vi "Save_Data.vi"(8 "error in (no error)":errorcluster, 11 "Message Queues out":T1) -> (0 "error out":errorcluster)   [LabVIEW 2023]
uses:
  Message Queue/All Message Queues.ctl
  Message Queue/Message Cluster.ctl
  controls/UI Data.ctl
  Drivers/Resideo Gas Valve/Type Definitions/Vesta Info.ctl
  Drivers/Resideo Gas Valve/Type Definitions/Temperature Control.ctl
  controls/Timer Application Cluster.ctl
  controls/Burner Duty Cycle.ctl
  Hybrid Water Heater/Type Definitions/HEWH MW100 Data Cluster.ctl
  Hybrid Water Heater/Custom Instrument Control/MW100/Type Definitions/HEWH Module 4 Relay Status.ctl
  Message Queue/Enqueue Message (Single).vi
  Message Queue/Message Queue.lvlib
panel:
  in  "Debug":bool
  out "Debug":string[](array[string])
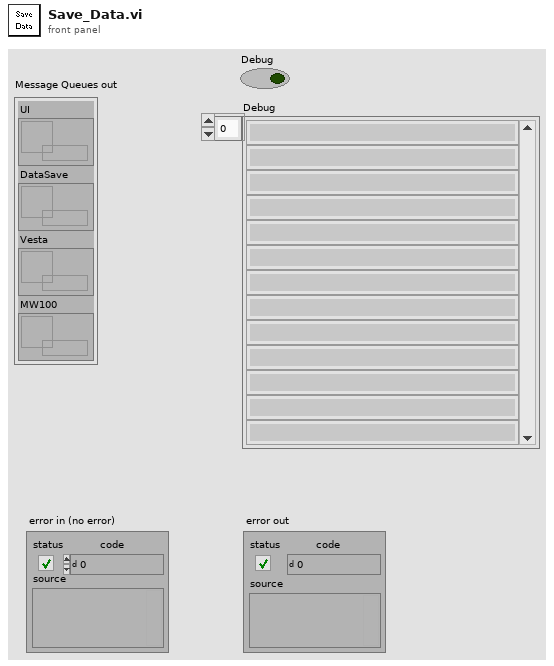
[diagram p1: front panel]
types:
  T1 = typedef "Message Queue.lvlib/All Message Queues.ctl" = cluster{"UI":refnum<queue>, "DataSave":refnum<queue>, "Vesta":refnum<queue>, "MW100":refnum<queue>}
  T2 = typedef "UI Data.ctl" = cluster{"Vesta Data Output":T3, "VestaTemperature":T4, "Timer Application Data":T5, "Data Array":string[][], "MW Output":T7}
  T3 = typedef "Vesta Info.ctl" = cluster{"Temp_W_Raw_U":u16, "Temp_W_Raw_L":u16, "Temperature Water (F)":dbl, "Temperature Water Compensated (F)":dbl, "Temperature Ambient (F)":dbl, "Setpoint Location (F)":dbl, "Heat Request":string, "Fault Ram":string, "PWM DCDC Value":u16, "Pilot Voltage (mV)":dbl, "Setpoint Actual (F)":dbl, "Differential Actual (F)":dbl, "Setpoint User (F)":dbl, "Differential User (F)":dbl, "Termperature FIltered -TCO (F)":dbl, "Temp_C_Raw_1 - Sensor Voltage":string, "Temp_C_Raw_2 - Sensor Voltage":string, "Chamber Sensor Temperature (F)":dbl, "LDO Base Temperature (F)":dbl, "LDO Timer (sec)":i16, "Disabled (0)":bool, "Warming (1)":bool, "Heating (2)":bool, "Cooling Data Write (3)":bool, "Cooling (4)":bool, "Data Read (5)":bool, "N/A":bool, "Temperature Trip (7)":bool, "Burner":bool}
  T4 = typedef "Temperature Control.ctl" = cluster{"Water Heater Temp (°F)":u16, "Differential  (°F)":dbl}
  T5 = typedef "Timer Application Cluster.ctl" = cluster{"Duty Cycle":T6}
  T6 = typedef "Burner Duty Cycle.ctl" = cluster{"Burner ON Time (Seconds)":dbl, "Burner OFF Time (Seconds)":dbl, "Main Burner Flag":bool, "Burner Power Mode":u8}
  T7 = typedef "HEWH MW100 Data Cluster.ctl" = cluster{"TC1-Channel 021":dbl, "TC2-Channel 022":dbl, "TC3-Channel 023":dbl, "TC4-Channel 024":dbl, "TC5-Channel 025":dbl, "TC6-Channel 026":dbl, "TC7-Channel 017":dbl, "TC8-Channel 028":dbl, "TC9-Channel 029":dbl, "TC10-Channel 030":dbl, "TC Tree Average":dbl, "TC DWN- Channel 027":dbl, "RTDin-Channel 031":dbl, "RTDout-Channel 032":dbl, "RTDamb-Channel 033":dbl, "PSI1-Channel 011":dbl, "PSI2-Channel 012":dbl, "PSI3-Channel 013":dbl, "PSI4-Channel 014":dbl, "UE State-Channel 015":dbl, "LE State-Channel 016":dbl, "Module 4 Relay Status Output":T8}
  T8 = typedef "HEWH Module 4 Relay Status.ctl" = cluster{"INTELLIFAUCET TEMP(T)/FLOW(F) (CH 041)":bool, "INTELLIFAUCET READY (CH 042)":bool, "INTELLIFAUCET START (CH 043)":bool, "INTELLIFAUCET STOP (CH 044)":bool, "MAIN POWER RELAY (CH 047)":bool, "NOT USED (CH 045)":bool, "NOT USED (CH 046)":bool, "PURGE VALVE RELAY (CH 048)":bool, "OUTLET VALVE RELAY (CH 049)":bool, "INLET VALVE RELAY (CH 050)":bool, "Intellifaucet (% Open)":dbl, "Proportioning Valve (%Open)":dbl, "Intellifaucet Temp Setpoint (F)":dbl}
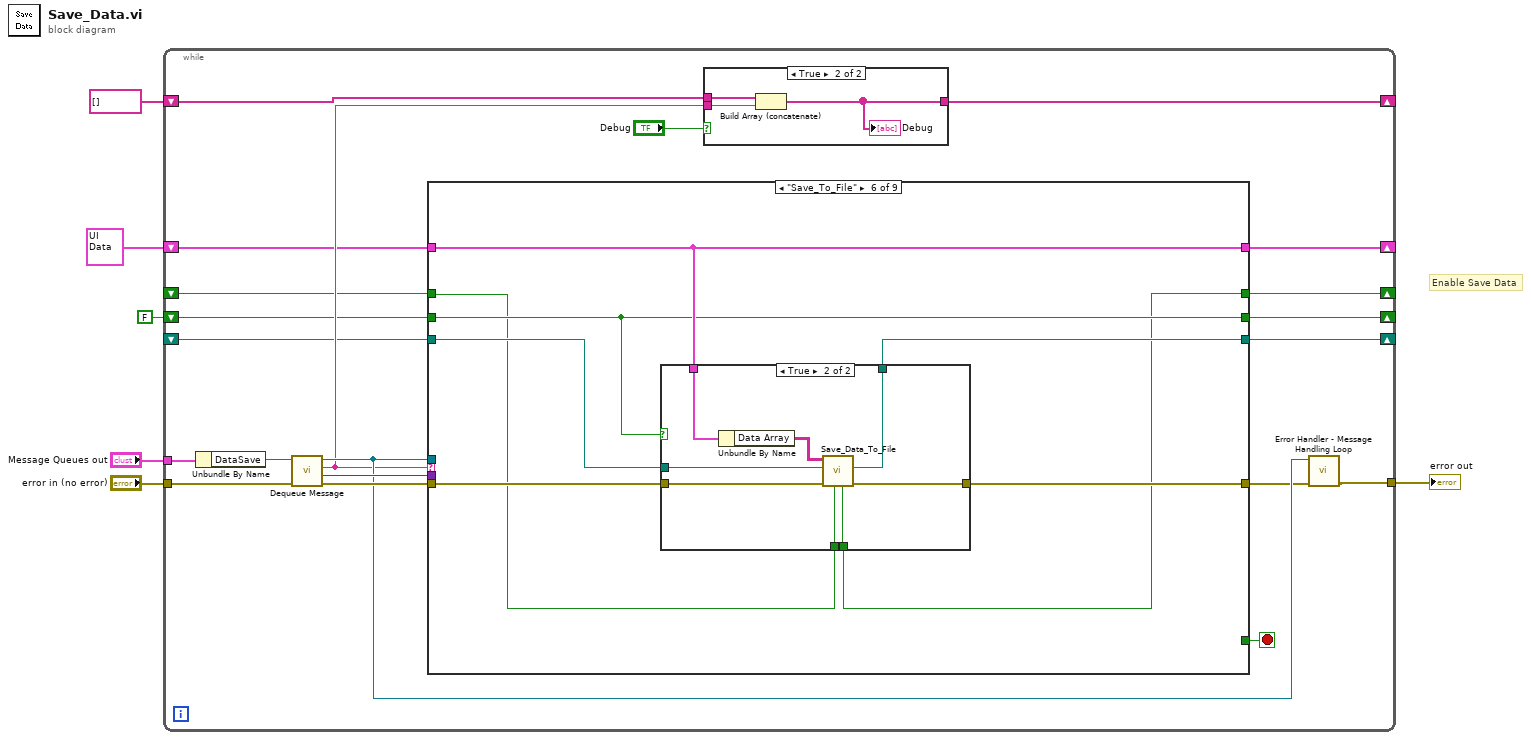
[diagram p0: block diagram]
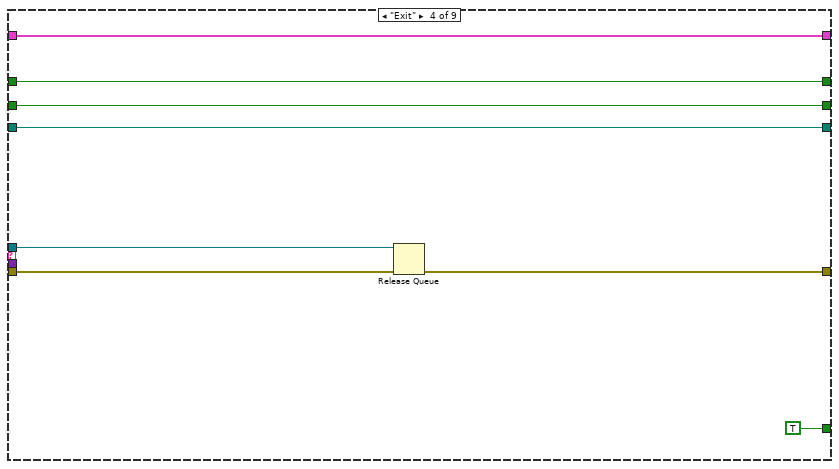
[diagram p6: hidden frame]
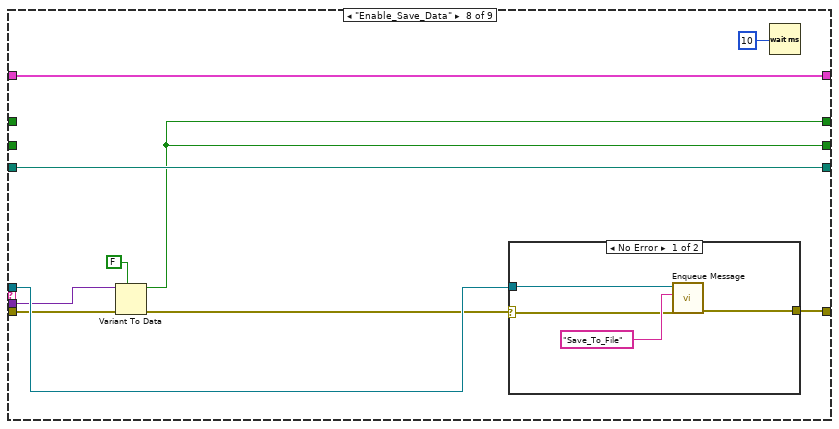
[diagram p10: hidden frame]
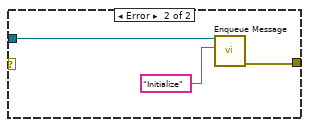
[diagram p11: hidden frame]
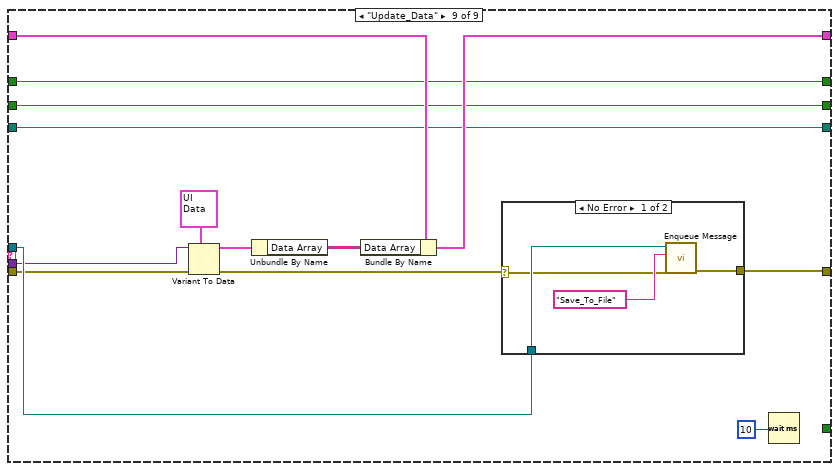
[diagram p12: hidden frame]
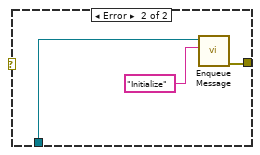
[diagram p13: hidden frame]
diagram:
  # "Enable Save Data"
  n1 = while {
    tunnel: "Message Queues out" -> [w20]
    tunnel: "error in (no error)" -> [w24]
    tunnel: [w17] -> w3
    shift-right: [w21] -> _
    shift-left: string[] [] -> [w22]
    shift-right: [w13] -> _
    shift-left: T2 {"Vesta Data Output"={"Temp_W_Raw_U"=0, "Temp_W_Raw_L"=0, "Temperature Water (F)"=0.0, "Temperature Water Compensated (F)"=0.0, "Temperature Ambient (F)"=0.0, "Setpoint Location (F)"=0.0, "Heat Request"="", "Fault Ram"="", "PWM DCDC Value"=0, "Pilot Voltage (mV)"=0.0, "Setpoint Actual (F)"=0.0, "Differential Actual (F)"=0.0, "Setpoint User (F)"=0.0, "Differential User (F)"=0.0, "Termperature FIltered -TCO (F)"=0.0, "Temp_C_Raw_1 - Sensor Voltage"="", "Temp_C_Raw_2 - Sensor Voltage"="", "Chamber Sensor Temperature (F)"=0.0, "LDO Base Temperature (F)"=0.0, "LDO Timer (sec)"=0, "Disabled (0)"=FALSE, "Warming (1)"=FALSE, "Heating (2)"=FALSE, "Cooling Data Write (3)"=FALSE, "Cooling (4)"=FALSE, "Data Read (5)"=FALSE, "N/A"=FALSE, "Temperature Trip (7)"=FALSE, "Burner"=FALSE}, "VestaTemperature"={"Water Heater Temp (°F)"=135, "Differential  (°F)"=10.0}, "Timer Application Data"={"Duty Cycle"={"Burner ON Time (Seconds)"=60.0, "Burner OFF Time (Seconds)"=60.0, "Main Burner Flag"=FALSE, "Burner Power Mode"=0}}, "Data Array"=[], "MW Output"={"TC1-Channel 021"=0.0, "TC2-Channel 022"=0.0, "TC3-Channel 023"=0.0, "TC4-Channel 024"=0.0, "TC5-Channel 025"=0.0, "TC6-Channel 026"=0.0, "TC7-Channel 017"=0.0, "TC8-Channel 028"=0.0, "TC9-Channel 029"=0.0, "TC10-Channel 030"=0.0, "TC Tree Average"=0.0, "TC DWN- Channel 027"=0.0, "RTDin-Channel 031"=0.0, "RTDout-Channel 032"=0.0, "RTDamb-Channel 033"=0.0, "PSI1-Channel 011"=0.0, "PSI2-Channel 012"=0.0, "PSI3-Channel 013"=0.0, "PSI4-Channel 014"=0.0, "UE State-Channel 015"=0.0, "LE State-Channel 016"=0.0, "Module 4 Relay Status Output"={"INTELLIFAUCET TEMP(T)/FLOW(F) (CH 041)"=FALSE, "INTELLIFAUCET READY (CH 042)"=FALSE, "INTELLIFAUCET START (CH 043)"=FALSE, "INTELLIFAUCET STOP (CH 044)"=FALSE, "MAIN POWER RELAY (CH 047)"=FALSE, "NOT USED (CH 045)"=FALSE, "NOT USED (CH 046)"=FALSE, "PURGE VALVE RELAY (CH 048)"=FALSE, "OUTLET VALVE RELAY (CH 049)"=FALSE, "INLET VALVE RELAY (CH 050)"=FALSE, "Intellifaucet (% Open)"=0.0, "Proportioning Valve (%Open)"=0.0, "Intellifaucet Temp Setpoint (F)"=0.0}}} ("Data Cluster Output") -> [w14]
    shift-right: [w12] -> _
    shift-left: FALSE -> [w11]
    shift-right: [w10] -> _
    shift-left: _ -> [w9]
    shift-right: [w8] -> _
    shift-left: _ -> [w7]
    stop <- w15 stop-if-true
    n2 = Unbundle By Name(w20) -> ("DataSave"=w27:refnum<queue>)
    n3 = call "Dequeue Message.vi"("error in (no error)"=w24, "Message Queue"=w27) -> ("error out"=w25:errorcluster, "Message Data"=w26:variant, "Message"=w16:string, "dup Message Queue"=w19:refnum<queue>)  [unwired: 6 in]
    n4 = case shown="\"Save_To_File\"" w16 {
      tunnel: w19 -> [_ _ _ w53 _ _ _ w92 w113]
      tunnel: w26 -> [_ _ _ _ _ _ _ w86 w109]
      tunnel: w25 -> [w36 w41 w44 w54 w59 w66 w83 w88 w111]
      tunnel: [w36 w41 w44 w52 w59 w65 w83 w93 w114] -> w18
      tunnel: [_ _ _ TRUE _ _ _ _ _] -> w15
      tunnel: w14 -> [w35 w40 w46 w50 w58 w67 w82 w90 w107]
      tunnel: [w35 w40 w46 w50 w58 w67 w82 w90 w106] -> w13
      tunnel: [w34 w39 w45 w49 w57 w62 w81 w84 w103] -> w12
      tunnel: w11 -> [w34 w39 w45 w49 w57 w62 w81 _ w103]
      tunnel: [w33 w38 w43 w48 w56 w64 w80 w85 w102] -> w10
      tunnel: w9 -> [w33 w38 w43 w48 w56 w63 w80 w85 w102]
      tunnel: [w32 w37 w42 w47 w55 w60 w79 w84 w101] -> w8
      tunnel: w7 -> [w32 w37 w42 w47 w55 w61 w79 _ w101]
      frame "---------- Setup ----------" {
      }
      frame Default {
      }
      frame "Initialize" {
      }
      frame "Exit" {
        n5 = Release Queue(queue=w53, error in (no error)=w54) -> (error out=w52:errorcluster)  [unwired: 1 in, 2 out]
      }
      frame "---------- Data Collection ----------" {
      }
      frame "Save_To_File" {
        n6 = case shown="True" w62 {
          tunnel: w67 -> [_ w78]
          tunnel: w66 -> [w69 w76]
          tunnel: [w69 w75] -> w65
          tunnel: [w70 w74] -> w64
          tunnel: w63 -> [w70 w73]
          tunnel: w61 -> [w68 w72]
          tunnel: [w68 w71] -> w60
          frame False {
          }
          frame True {
            n7 = Unbundle By Name(w78) -> ("Data Array"=w77:string[][])
            n8 = call "Save_Data_To_File.vi"("Save Header?"=w72, "error in (no error)"=w76, "Filepath Input"=w73, "Data Array in"=w77) -> ("error out"=w75:errorcluster, "Filepath Output"=w74:path, "Save Header Out?"=w71:bool)  [unwired: 5 in]
          }
        }
      }
      frame "---------- Save Control ----------" {
      }
      frame "Enable_Save_Data" {
        n9 = Variant To Data(error in=w88, type=FALSE, Variant=w86) -> (data=w84:bool, error out=w87:errorcluster)
        n10 = case shown="No Error" w87 {
          selector: w87 -> [w94 _]
          tunnel: [w96 w100] -> w93
          tunnel: w92 -> [w95 w98]
          frame No Error {
            n11 = call-poly "Enqueue Message.vi"("error in (no error)"=w94, "Message"="Save_To_File", "Message Queue"=w95) -> ("error out"=w96:errorcluster)  [unwired: 7 in, 1 out]
          }
          frame Error {
            n12 = call-poly "Enqueue Message.vi"("Message"="Initialize", "Message Queue"=w98) -> ("error out"=w100:errorcluster)  [unwired: 8 in, 1 out]
          }
        }
        n13 = Wait (ms)(milliseconds to wait=u32 10) -> ()  [unwired: 1 out]
      }
      frame "Update_Data" {
        n14 = Variant To Data(error in=w111, type=T2 {"Vesta Data Output"={"Temp_W_Raw_U"=0, "Temp_W_Raw_L"=0, "Temperature Water (F)"=0.0, "Temperature Water Compensated (F)"=0.0, "Temperature Ambient (F)"=0.0, "Setpoint Location (F)"=0.0, "Heat Request"="", "Fault Ram"="", "PWM DCDC Value"=0, "Pilot Voltage (mV)"=0.0, "Setpoint Actual (F)"=0.0, "Differential Actual (F)"=0.0, "Setpoint User (F)"=0.0, "Differential User (F)"=0.0, "Termperature FIltered -TCO (F)"=0.0, "Temp_C_Raw_1 - Sensor Voltage"="", "Temp_C_Raw_2 - Sensor Voltage"="", "Chamber Sensor Temperature (F)"=0.0, "LDO Base Temperature (F)"=0.0, "LDO Timer (sec)"=0, "Disabled (0)"=FALSE, "Warming (1)"=FALSE, "Heating (2)"=FALSE, "Cooling Data Write (3)"=FALSE, "Cooling (4)"=FALSE, "Data Read (5)"=FALSE, "N/A"=FALSE, "Temperature Trip (7)"=FALSE, "Burner"=FALSE}, "VestaTemperature"={"Water Heater Temp (°F)"=135, "Differential  (°F)"=10.0}, "Timer Application Data"={"Duty Cycle"={"Burner ON Time (Seconds)"=60.0, "Burner OFF Time (Seconds)"=60.0, "Main Burner Flag"=FALSE, "Burner Power Mode"=0}}, "Data Array"=[], "MW Output"={"TC1-Channel 021"=0.0, "TC2-Channel 022"=0.0, "TC3-Channel 023"=0.0, "TC4-Channel 024"=0.0, "TC5-Channel 025"=0.0, "TC6-Channel 026"=0.0, "TC7-Channel 017"=0.0, "TC8-Channel 028"=0.0, "TC9-Channel 029"=0.0, "TC10-Channel 030"=0.0, "TC Tree Average"=0.0, "TC DWN- Channel 027"=0.0, "RTDin-Channel 031"=0.0, "RTDout-Channel 032"=0.0, "RTDamb-Channel 033"=0.0, "PSI1-Channel 011"=0.0, "PSI2-Channel 012"=0.0, "PSI3-Channel 013"=0.0, "PSI4-Channel 014"=0.0, "UE State-Channel 015"=0.0, "LE State-Channel 016"=0.0, "Module 4 Relay Status Output"={"INTELLIFAUCET TEMP(T)/FLOW(F) (CH 041)"=FALSE, "INTELLIFAUCET READY (CH 042)"=FALSE, "INTELLIFAUCET START (CH 043)"=FALSE, "INTELLIFAUCET STOP (CH 044)"=FALSE, "MAIN POWER RELAY (CH 047)"=FALSE, "NOT USED (CH 045)"=FALSE, "NOT USED (CH 046)"=FALSE, "PURGE VALVE RELAY (CH 048)"=FALSE, "OUTLET VALVE RELAY (CH 049)"=FALSE, "INLET VALVE RELAY (CH 050)"=FALSE, "Intellifaucet (% Open)"=0.0, "Proportioning Valve (%Open)"=0.0, "Intellifaucet Temp Setpoint (F)"=0.0}}} ("Data Cluster Output 2"), Variant=w109) -> (data=w105:T2, error out=w110:errorcluster)
        n15 = Unbundle By Name(w105) -> ("Data Array"=w104:string[][])
        n16 = Bundle By Name(cluster=w107, "Data Array"=w104) -> (w106:T2)
        n17 = case shown="No Error" w110 {
          selector: w110 -> [w115 _]
          tunnel: [w117 w121] -> w114
          tunnel: w113 -> [w116 w119]
          frame No Error {
            n18 = call-poly "Enqueue Message.vi"("error in (no error)"=w115, "Message"="Save_To_File", "Message Queue"=w116) -> ("error out"=w117:errorcluster)  [unwired: 7 in, 1 out]
          }
          frame Error {
            n19 = call-poly "Enqueue Message.vi"("Message"="Initialize", "Message Queue"=w119) -> ("error out"=w121:errorcluster)  [unwired: 8 in, 1 out]
          }
        }
        n20 = Wait (ms)(milliseconds to wait=u32 10) -> ()  [unwired: 1 out]
      }
    }
    n21 = case shown="True" "Debug" {
      tunnel: w16 -> [_ w31]
      tunnel: w22 -> [w28 w30]
      tunnel: [w28 w29] -> w21
      frame False {
      }
      frame True {
        n22 = Build Array (concatenate)(w30, w31) -> (w29:string[])
        "Debug" <- w29
      }
    }
    n23 = call "Error Handler - Message Handling Loop.vi"("error in (no error)"=w18, "Message Queue"=w19) -> ("dup error in"=w17:errorcluster)  [unwired: 8 in, 1 out]
  }
  "error out" <- w3
